vi "Background Process Directors.vi"(8 "error in (no error)":errorcluster, 9 "Results Notifier":refnum<notifier>, 10 "Wait Time":u32 caption="ms" step=1, 11 "InteractionProcessor in":refnum<class "InteractionProcessor.lvclass">) -> (0 "error out":errorcluster, 3 "InteractionProcessor out":refnum<class "InteractionProcessor.lvclass">)   [LabVIEW 2023, in "HAF.lvlib" / "InteractionProcessor.lvclass"]
doc: "Calls the Process Directors method asynchronously, without waiting for a result (Process Director notifies results.)  Using this approach means the User Test Application UI isn’t blocked by long-running Commands and can remain responsive to result notifications."
uses:
  InteractionProcessor.lvclass
  ReadCommand/ReadCommand.lvclass
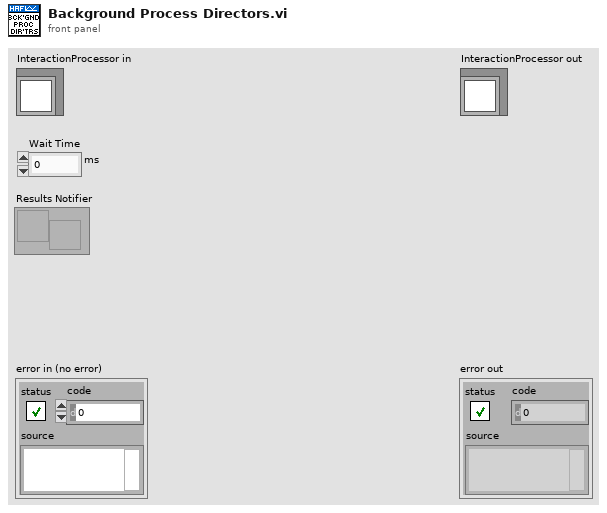
[diagram p1: front panel]
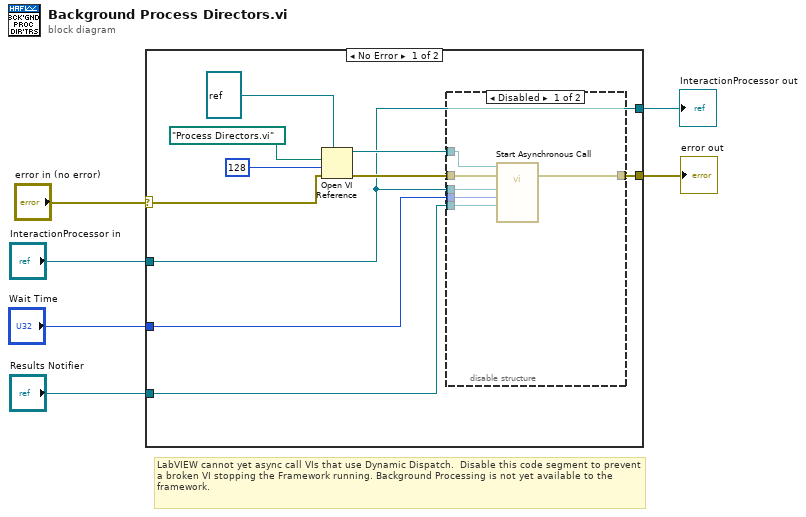
[diagram p0: block diagram]
diagram:
  # "LabVIEW cannot yet async call VIs that use Dynamic Dispatch.  Disable this code segment to prevent a broken VI stopping the Framework running. Background Processing is not yet available to the framework."
  n1 = case shown="No Error" "error in (no error)" {
    selector: "error in (no error)" -> [w16 w24]
    tunnel: [w7 w24] -> w5
    tunnel: [w8 w23] -> w3
    tunnel: "InteractionProcessor in" -> [w8 w23]
    tunnel: "Wait Time" -> [w11 _]
    tunnel: "Results Notifier" -> [w10 _]
    frame No Error {
      n2 = Open VI Reference(type specifier VI Refnum (for type only)=refnum<vi> refnum, vi path=path "Process Directors.vi", options=128, error in (no error)=w16) -> (vi reference=w13:refnum<vi>, error out=w9:errorcluster)  [unwired: 2 in]
      n3 = disable-structure shown="Disabled" {
        disable-tunnel: w13 -> [w22 _]
        disable-tunnel: w11 -> [w21 _]
        disable-tunnel: w10 -> [w20 _]
        disable-tunnel: w9 -> [w19 _]
        disable-tunnel: w8 -> [w18 _]
        disable-tunnel: [w17 _] -> w7
        frame Disabled {
          n4 = call-by-ref "Start Asynchronous Call"(reference=w22, error in=w19, "Results Notifier"=w20, "Wait Time"=w21, "TestProcessor in"=w18) -> (error out=w17:errorcluster)  [unwired: 7 in, 3 out]
        }
        frame Enabled {
        }
      }
    }
    frame Error {
    }
  }
  "error out" <- w5
  "InteractionProcessor out" <- w3
